vi "Main Page.vi"(8 "error in (no error)":errorcluster, 11 "Node Ptr":T1 format="%.0x") -> (0 "error out":errorcluster)   [LabVIEW 2017, in "DSF System Explorer.lvlib"]
uses:
  DSF System Explorer.lvlib
  <vilib>/NI Veristand/Custom Device API/Custom Device Item Ref.ctl
  <vilib>/NI Veristand/Custom Device API/Custom Device API.lvlib
panel:
  in  "refresh config":bool
  in  "open_config_viewer":bool
  in  "DSF Configuration Path":path
  in  "Header":cluster{"Section Name":string}={"Section Name"="Custom Device Item Settings"}
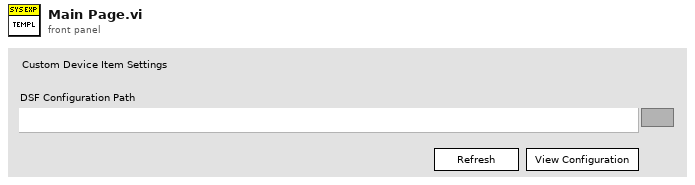
[diagram p1: front panel]
types:
  T1 = typedef "Custom Device API.lvlib/Custom Device Item Ref.ctl" = u64
  T2 = typedef "Custom Device API.lvlib/Custom Device Commands.ctl" = enum16{"Default", "Item renamed", "Shutdown", "Dynamic button pressed"}
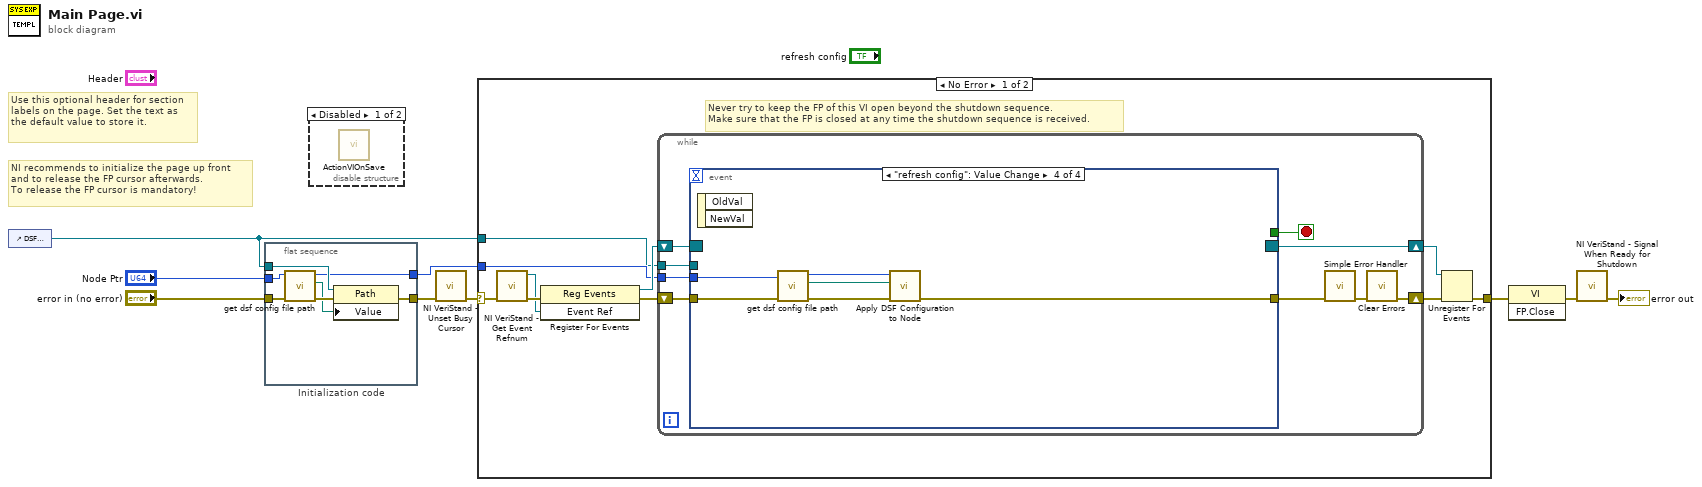
[diagram p0: block diagram]
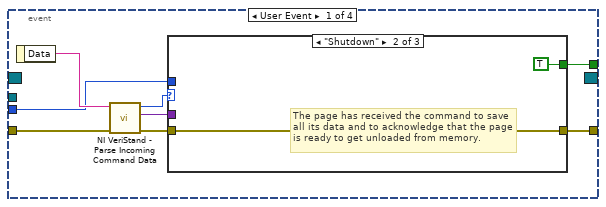
[diagram p3: hidden frame]
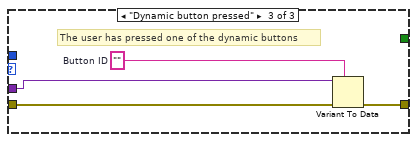
[diagram p5: hidden frame]
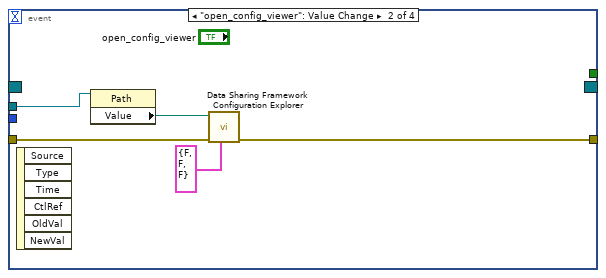
[diagram p6: hidden frame]
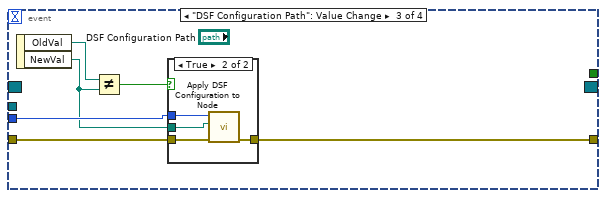
[diagram p7: hidden frame]
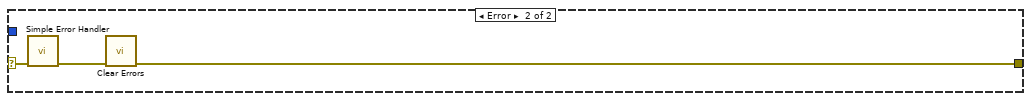
[diagram p9: hidden frame]
diagram:
  # "Use this optional header for section labels on the page. Set the text as the default value to store it."
  # "NI recommends to initialize the page up front\nand to release the FP cursor afterwards.\nTo release the FP cursor is mandatory!"
  n1 = control-ref of="DSF Configuration Path"() -> (w1:refnum<vi>)
  n2 = flat-sequence "Initialization code" {
    tunnel: "error in (no error)" -> [w15]
    tunnel: "Node Ptr" -> [w16]
    tunnel: [w13] -> w5
    tunnel: [w11] -> w2
    tunnel: w1 -> [w12]
    frame #0 {
      n3 = call "get dsf config file path.vi"("error in (no error)"=w15, "Node Ptr"=w16) -> ("error out"=w14:errorcluster, "Path"=w10:path, "Item Ref out"=w11:T1)  [unwired: 7 in]
      n4 = property class="Path"(reference=w12, error in=w14, "Value"=w10) -> (error out=w13:errorcluster)  [unwired: 1 out]
    }
  }
  n5 = disable-structure shown="Disabled" {
    frame Disabled {
      n6 = call "ActionVIOnSave.vi"() -> ()  [unwired: 10 in, 2 out]
    }
    frame Enabled {
    }
  }
  n7 = call <vilib>:"NI VeriStand - Unset Busy Cursor.vi"("error in (no error)"=w5) -> ("error out"=w4:errorcluster)  [unwired: 10 out]
  n8 = case shown="No Error" w4 {
    selector: w4 -> [w18 w75]
    tunnel: [w23 w73] -> w9
    tunnel: w2 -> [w19 _]
    tunnel: w1 -> [w17 _]
    frame No Error {
      # "Never try to keep the FP of this VI open beyond the shutdown sequence.\nMake sure that the FP is closed at any time the shutdown sequence is received."
      n9 = call <vilib>:"NI VeriStand - Get Event Refnum.vi"("error in (no error)"=w18) -> ("error out"=w26:errorcluster, "Event Ref"=w22:refnum<user-event>)  [unwired: 9 out]
      n10 = register-events(error in=w26, w22) -> (reference out=w20:refnum<event-registration>, error out=w21:errorcluster)  [unwired: 1 in]
      n11 = while {
        tunnel: w19 -> [w31]
        shift-right: [w28] -> w24
        shift-left: w21 -> [w34]
        shift-right: [w35] -> w25
        shift-left: w20 -> [w33]
        tunnel: w17 -> [w27]
        stop <- w32 stop-if-true
        n12 = event shown="[3] \"refresh config\": Value Change" {
          selector: w33 -> [_ _ _ _]
          dyn-events: [_ _ _ _] -> w35
          timeout: _ -> [_ _ _ _]
          tunnel: w34 -> [w43 w55 w61 w72]
          tunnel: [w39 _ _ _] -> w32
          tunnel: [w38 w54 w59 w67] -> w30
          tunnel: w31 -> [w37 _ w60 w70]
          tunnel: w27 -> [_ w53 _ _]
          event User Event {
            n13 = event-data() -> ("Data"=w42:string)  [unwired: 1 out]
            n14 = call <vilib>:"NI VeriStand - Parse Incoming Command Data.vi"("error in (no error)"=w43, "Incoming data"=w42) -> ("error out"=w41:errorcluster, "Outgoing data"=w36:variant, "Action"=w40:T2)  [unwired: 7 out]
            n15 = case shown="\"Shutdown\"" w40 {
              tunnel: w41 -> [w44 w45 w50]
              tunnel: [_ TRUE _] -> w39
              tunnel: [w44 w45 w47] -> w38
              tunnel: w37 -> [_ _ _]
              tunnel: w36 -> [_ _ w49]
              frame "Default", Default {
              }
              frame "Shutdown" {
                # "The page has received the command to save all its data and to acknowledge that the page is ready to get unloaded from memory."
              }
              frame "Dynamic button pressed" {
                w48 = ""  # Button ID
                # "The user has pressed one of the dynamic buttons"
                n16 = Variant To Data(error in=w50, type=w48, Variant=w49) -> (error out=w47:errorcluster)  [unwired: 1 out]
              }
            }
          }
          event "open_config_viewer": Value Change {
            n17 = event-data() -> ()  [unwired: 7 out]
            n18 = property class="Path"(reference=w53) -> ("Value"=w52:path)  [unwired: 1 in, 2 out]
            n19 = call "Data Sharing Framework Configuration Explorer.vi"("menu options"=cluster{"open":bool, "save":bool, "view":bool} {"open"=FALSE, "save"=FALSE, "view"=FALSE}, "error in (no error)"=w55, "Path in"=w52) -> ("error out"=w54:errorcluster)  [unwired: 7 in, 1 out]
          }
          event "DSF Configuration Path": Value Change {
            n20 = event-data() -> ("OldVal"=w58:path, "NewVal"=w57:path)  [unwired: 1 out]
            n21 = Not Equal?(x=w58, y=w57) -> (x != y?=w56:bool)
            n22 = case shown="True" w56 {
              tunnel: w61 -> [w62 w66]
              tunnel: w60 -> [_ w63]
              tunnel: [w62 w65] -> w59
              tunnel: w57 -> [_ w64]
              frame False {
              }
              frame True {
                n23 = call "Apply DSF Configuration to Node.vi"("error in (no error)"=w66, "NewVal"=w64, "Item Ref in"=w63) -> ("error out"=w65:errorcluster)  [unwired: 8 in]
              }
            }
          }
          event "refresh config": Value Change {
            n24 = event-data() -> ()  [unwired: 3 out]
            n25 = call "get dsf config file path.vi"("error in (no error)"=w72, "Node Ptr"=w70) -> ("error out"=w71:errorcluster, "Path"=w68:path, "Item Ref out"=w69:T1)  [unwired: 7 in]
            n26 = call "Apply DSF Configuration to Node.vi"("error in (no error)"=w71, "NewVal"=w68, "Item Ref in"=w69) -> ("error out"=w67:errorcluster)  [unwired: 8 in]
          }
        }
        n27 = call <vilib>:"Simple Error Handler.vi"("error in (no error)"=w30) -> ("error out"=w29:errorcluster)  [unwired: 1 in, 7 out]
        n28 = call <vilib>:"Clear Errors.vi"("error in (no error)"=w29) -> ("error out"=w28:errorcluster)  [unwired: 1 in, 5 out]
      }
      n29 = Unregister For Events(event registration refnum=w25, error in=w24) -> (error out=w23:errorcluster)
    }
    frame Error {
      n30 = call <vilib>:"Simple Error Handler.vi"("error in (no error)"=w75) -> ("error out"=w74:errorcluster)  [unwired: 1 in, 7 out]
      n31 = call <vilib>:"Clear Errors.vi"("error in (no error)"=w74) -> ("error out"=w73:errorcluster)  [unwired: 1 in, 5 out]
    }
  }
  n32 = invoke class="VI" method="FP.Close"(error in=w9) -> (error out=w8:errorcluster)  [unwired: 2 in, 2 out]
  n33 = call <vilib>:"NI VeriStand - Signal When Ready for Shutdown.vi"("error in (no error)"=w8) -> ("error out"=→"error out":errorcluster)  [unwired: 10 out]
